vi "test_Format Debug String_Version and Name.vi"(8 "error in (no error)":errorcluster, 11 "TestCase in":refnum<class "Instrument Addon Unit Tests.lvclass">) -> (0 "error out":errorcluster, 3 "TestCase out":refnum<class "Instrument Addon Unit Tests.lvclass">)   [LabVIEW 2020, in "Instrument Addon Unit Tests.lvclass"]
uses:
  Instrument Addon Unit Tests.lvclass
  <vilib>/Utility/SystemLogging/Write to System Log.vi
  <vilib>/addons/_JKI Toolkits/VI Tester/TestCase.llb/TestCase.lvclass
  Addon/Addon Engine/Instrument Addon Engine.lvlib
  C:/Program Files (x86)/National Instruments/LabVIEW 2020/vi.lib/addons/_JKI Toolkits/VI Tester/TestCase.llb/TestCase.lvclass
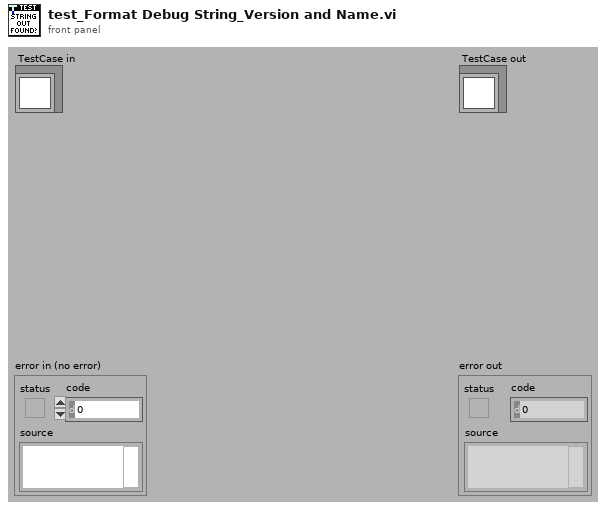
[diagram p1: front panel]
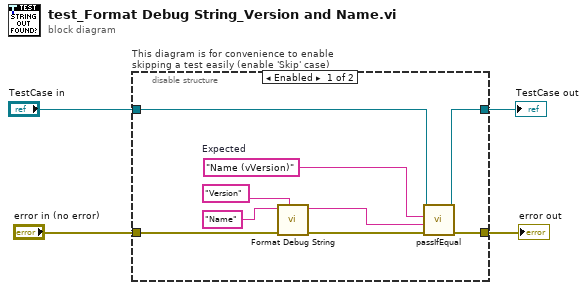
[diagram p0: block diagram]
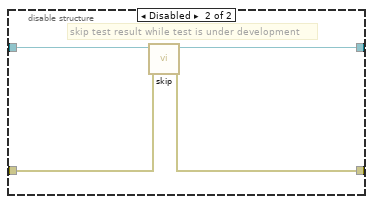
[diagram p2: hidden frame]
diagram:
  n1 = disable-structure "This diagram is for convenience to enable skipping a test easily (enable 'Skip' case)" shown="Enabled" {
    disable-tunnel: "TestCase in" -> [w11 w17]
    disable-tunnel: [w12 w15] -> w1
    disable-tunnel: [w13 w16] -> w3
    disable-tunnel: "error in (no error)" -> [w8 w14]
    frame Enabled {
      w6 = "Name (vVersion)"  # Expected
      n2 = call "Format Debug String.vi"("Version"="Version", "error in (no error)"=w8, "Name"="Name") -> ("error out"=w7:errorcluster, "Debug String"=w10:string)  [unwired: 7 in]
      n3 = call-dynamic "passIfEqual.vi"("error in (no error)"=w7, "y"=w10, "x"=w6, "TestCase in"=w11) -> ("error out"=w13:errorcluster, "TestCase out"=w12:refnum<class "Instrument Addon Unit Tests.lvclass">)  [unwired: 6 in]
    }
    frame Disabled {
      # "skip test result while test is under development"
      n4 = call <vilib>:"skip.vi"("error in (no error)"=w14, "TestCase in"=w17) -> ("error out"=w16:errorcluster, "TestCase out"=w15:refnum<class "Instrument Addon Unit Tests.lvclass">)  [unwired: 8 in]
    }
  }
  "error out" <- w3
  "TestCase out" <- w1
